vi "Software Update HCC Update INI File.vi"(11 "Path":path) -> ()   [LabVIEW 2016]
uses:
  <vilib>/Utility/file.llb/Read Delimited Spreadsheet (string).vi
  <vilib>/Utility/file.llb/Write Delimited Spreadsheet (string).vi
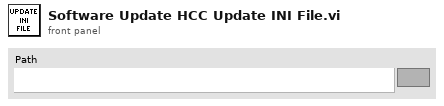
[diagram p1: front panel]
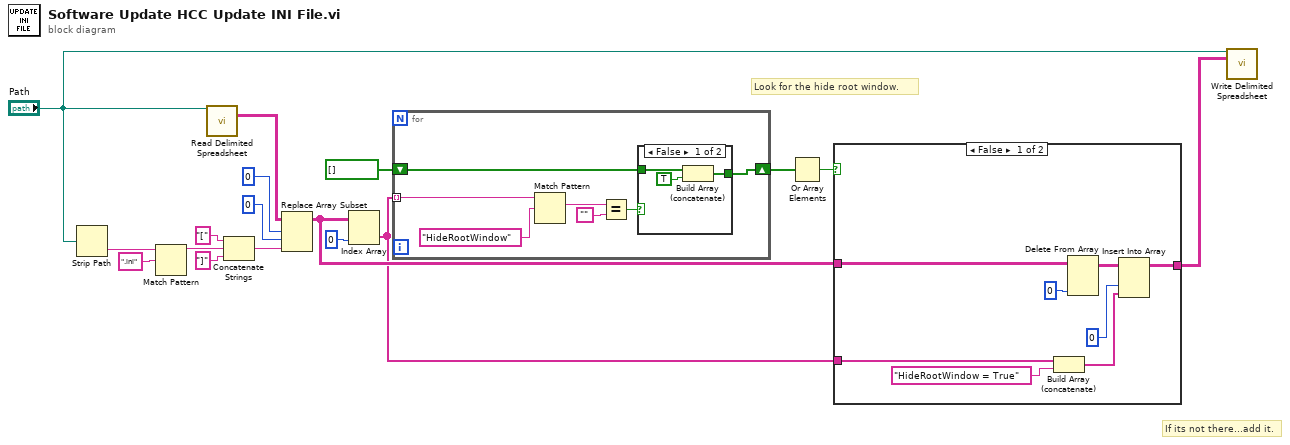
[diagram p0: block diagram]
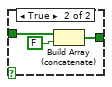
[diagram p3: hidden frame]
diagram:
  # "If its not there...add it."
  # "Look for the hide root window."
  n1 = Strip Path(path="Path") -> (name=w11:string)  [unwired: 1 out]
  n2 = Match Pattern(string=w11, regular expression=".ini") -> (before substring=w14:string)  [unwired: 1 in, 3 out]
  n3 = call-poly <vilib>:"Read Delimited Spreadsheet.vi"("file path (dialog if empty)"="Path") -> ("all rows"=w3:string[][])  [unwired: 9 in, 5 out]
  n4 = Concatenate Strings("[" ("string"), w14, "]" ("string")) -> (w17:string)
  n5 = Replace Array Subset(array=w3, new element=w17, index (row)=0, index (col)=0 ("disabled index (col)")) -> (w5:string[][])
  n6 = Index Array(array=w5, index (col)=0 ("disabled index (col)")) -> (element=w4:string[])  [unwired: 1 in]
  n7 = for {
    tunnel: w4 -> [w24] mode=indexing
    shift-right: [w21] -> w7
    shift-left: bool[] [] -> [w22]
    n8 = Match Pattern(string=w24, regular expression="HideRootWindow") -> (match substring=w20:string)  [unwired: 1 in, 3 out]
    n9 = Equal?(x=w20, y="") -> (x = y?=w18:bool)
    n10 = case shown="False" w18 {
      tunnel: w22 -> [w26 w30]
      tunnel: [w25 w29] -> w21
      frame False {
        n11 = Build Array (concatenate)(w26, TRUE) -> (w25:bool[])
      }
      frame True {
        n12 = Build Array (concatenate)(w30, FALSE) -> (w29:bool[])
      }
    }
  }
  n13 = Or Array Elements(Boolean array=w7) -> (logical OR=w6:bool)
  n14 = case shown="False" w6 {
    tunnel: w5 -> [w36 w39]
    tunnel: w4 -> [w37 _]
    tunnel: [w31 w39] -> w1
    frame False {
      n15 = Build Array (concatenate)(w37, "HideRootWindow = True") -> (w33:string[])
      n16 = Delete From Array(array=w36, index (col)=0 ("disabled index (col)")) -> (array with subset deleted=w34:string[][])  [unwired: 2 in, 1 out]
      n17 = Insert Into Array(array=w34, index (col)=0 ("disabled index (col)"), new element=w33) -> (w31:string[][])  [unwired: 1 in]
    }
    frame True {
    }
  }
  n18 = call-poly <vilib>:"Write Delimited Spreadsheet.vi"("file path (dialog if empty)"="Path", "2D data"=w1) -> ()  [unwired: 12 in, 2 out]
